vi "Get SMO Name.vi"(8 "error in (no error)":errorcluster, 11 "Instrument.Lockin":refnum<class "Instrument.Lockin.lvclass">) -> (0 "error out":errorcluster, 2 "SMO Name":string, 3 "Instrument.Lockin out":refnum<class "Instrument.Lockin.lvclass">)   [LabVIEW 2019, in "Instrument.Lockin.lvclass"]
uses:
  Instrument.Lockin.lvclass
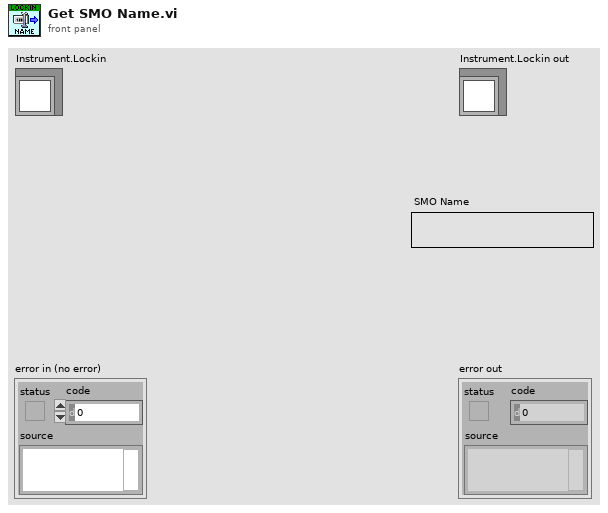
[diagram p1: front panel]
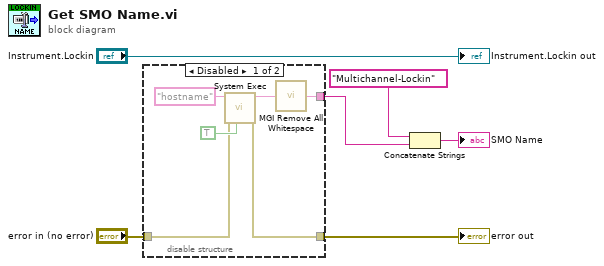
[diagram p0: block diagram]
diagram:
  n1 = disable-structure shown="Disabled" {
    disable-tunnel: "error in (no error)" -> [w8 w13]
    disable-tunnel: [w7 w13] -> w3
    disable-tunnel: [w9 _] -> w2
    frame Disabled {
      n2 = call <vilib>:"System Exec.vi"("run minimized? (F)"=TRUE, "error in (no error)"=w8, "command line"="hostname") -> ("error out"=w7:errorcluster, "standard output"=w10:string)  [unwired: 5 in, 2 out]
      n3 = call <userlib>:"MGI Remove All Whitespace.vi"("String"=w10) -> ("Trimmed String"=w9:string)
    }
    frame Enabled {
    }
  }
  "error out" <- w3
  n4 = Concatenate Strings("Multichannel-Lockin" ("SMO Name"), w2) -> (→"SMO Name":string)
  "Instrument.Lockin out" <- "Instrument.Lockin"
